vi "mqttFlagsRead.vi"(0 "mqtt in":refnum<class "mqtt.lvclass">, 11 "error in (no error)":errorcluster) -> (4 "mqtt out":refnum<class "mqtt.lvclass">, 6 "connFlags":T1, 15 "error out":errorcluster)   [LabVIEW 2013, in "mqtt.lvclass"]
uses:
  mqtt.lvclass
  mqttTypedef/mqttConnectionFlags.ctl
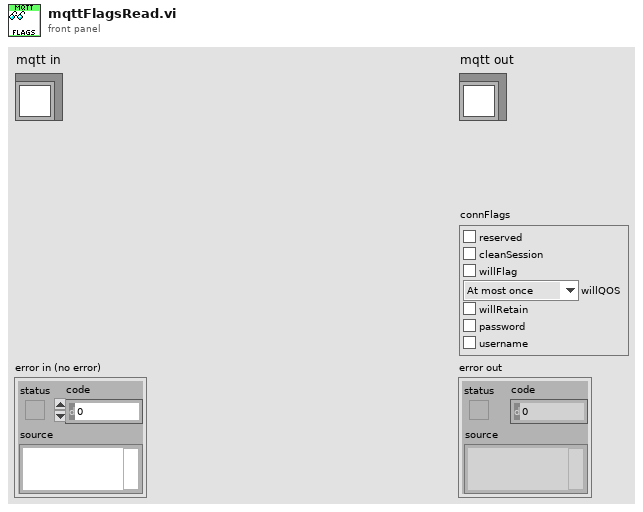
[diagram p1: front panel]
types:
  T1 = typedef "mqttConnectionFlags.ctl" = cluster{"reserved":bool, "clean session":bool, "will flag":bool, "willQOS":enum8{"At most once", "At least once", "Exactly once", "Reserved"}, "will retain":bool, "password":bool, "user name":bool}
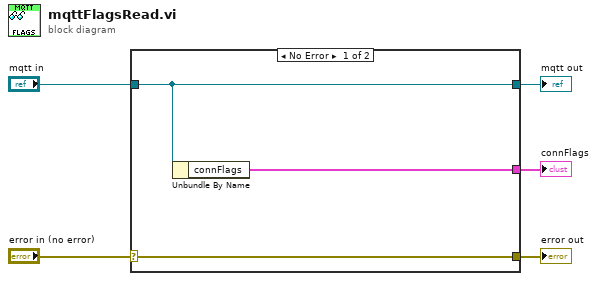
[diagram p0: block diagram]
diagram:
  n1 = case shown="No Error" "error in (no error)" {
    selector: "error in (no error)" -> [w8 w9]
    tunnel: [w8 w9] -> w4
    tunnel: [w7 w10] -> w2
    tunnel: "mqtt in" -> [w7 w10]
    tunnel: [w6 _] -> w1
    frame No Error {
      n2 = Unbundle By Name(w7) -> ("connFlags"=w6:T1)
    }
    frame Error {
    }
  }
  "error out" <- w4
  "mqtt out" <- w2
  "connFlags" <- w1
